vi "N Field Set Act.vi"(0 "command text in":string[](array[string]), 1 "Magnet":T1) -> ()   [LabVIEW 2025]
doc: "Author: Scott Hannahs <sth@magnet.fsu.edu>\n\nThis software is licensed for use under the “MIT License\"\nCopyright (c) 2025 Scott Hannahs, sth@sth@magnet.sthnet.net\n\nPermission is hereby granted, free of charge, to any person obtaining a copy of this software and associated documentation files (the \"Software\"), to deal in the Software without restriction, including without limitation the rights to use, copy, modify, merge, publish, distribute, sublicense, and/or sell copies of the Software, and to permit persons to whom the Software is furnished to do so, subject to the following conditions: The above copyright notice and this permission notice shall be included in all copies or substantial portions of the Software.\n\nTHE SOFTWARE IS PROVIDED \"AS IS\", WITHOUT WARRANTY OF ANY KIND, EXPRESS OR IMPLIED, INCLUDING BUT NOT LIMITED TO THE WARRANTIES OF MERCHANTABILITY, FITNESS FOR A PARTICULAR PURPOSE AND NONINFRINGEMENT. IN NO EVENT SHALL THE AUTHORS OR COPYRIGHT HOLDERS BE LIABLE FOR ANY CLAIM, DAMAGES OR OTHER LIABILITY, WHETHER IN AN ACTION OF CONTRACT, TORT OR OTHERWISE, ARISING FROM, OUT OF OR IN CONNECTION WITH THE SOFTWARE OR THE USE OR OTHER DEALINGS IN THE SOFTWARE."
uses:
  Ctl/magnet.ctl
  Which Power Supply.ctl
panel:
  out "error out 2":errorcluster
  out "error out":errorcluster
  in  "extra wait (sec)":i32
  in  "Rate":dbl
  in  "Field Set":dbl
  # "No wait"
  # "wait"
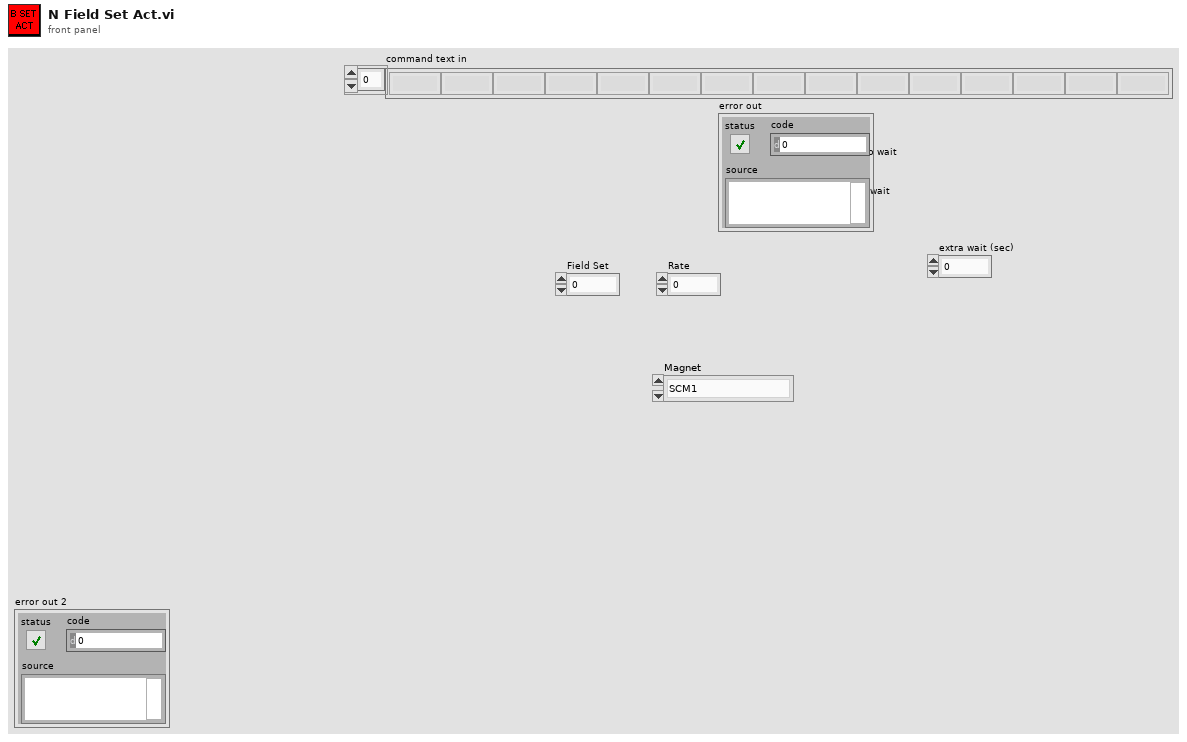
[diagram p1: front panel]
types:
  T1 = typedef "magnet.ctl" = enum16{"SCM1", "SCM2", "SCM3", "SCMX", "Cell8", "Cell9", "Cell12", "Hybrid", "Great Magnet"}
  T2 = typedef "Which Power Supply.ctl" = enum16{"Superconducting Magnet", "Resistive Magnet", "Hybrid Magnet"}
  T3 = typedef "Field Set.ctl" = cluster{"rate":dbl, "set point":dbl, "extra wait":i32, "wait option":u16}
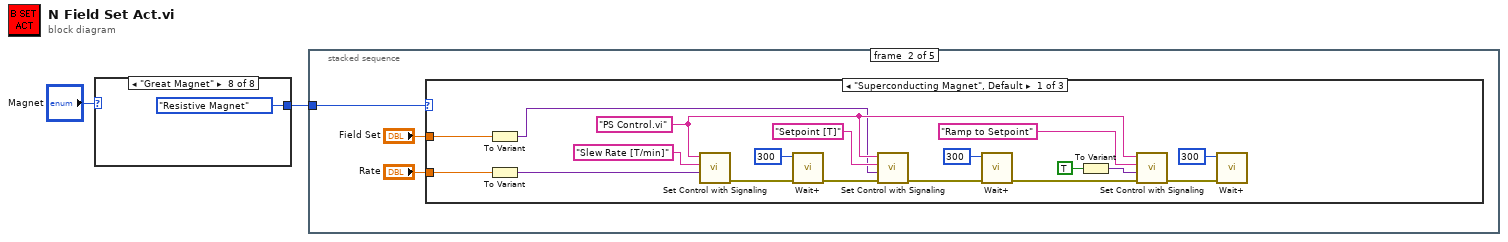
[diagram p0: block diagram]
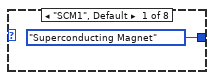
[diagram p2: hidden frame]
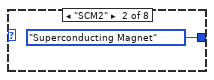
[diagram p3: hidden frame]
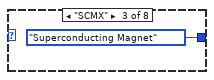
[diagram p4: hidden frame]
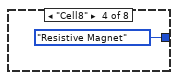
[diagram p5: hidden frame]
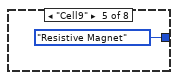
[diagram p6: hidden frame]
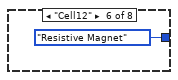
[diagram p7: hidden frame]
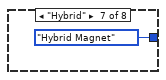
[diagram p8: hidden frame]
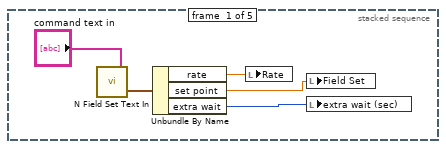
[diagram p9: hidden frame]
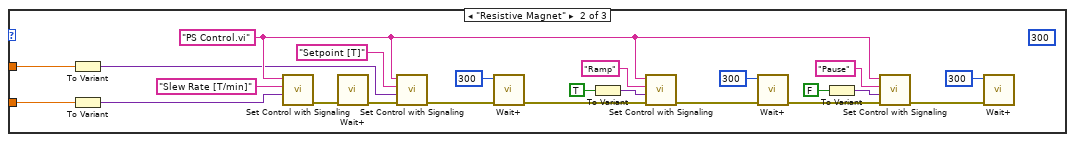
[diagram p10: hidden frame]
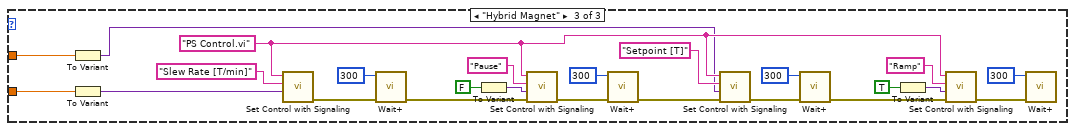
[diagram p11: hidden frame]
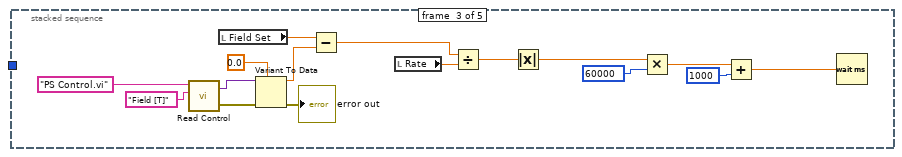
[diagram p12: hidden frame]
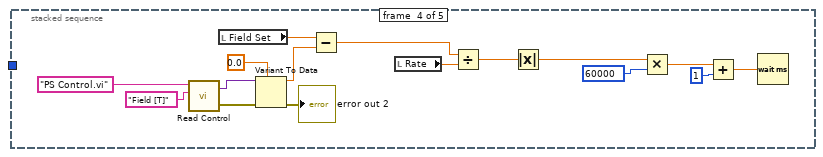
[diagram p13: hidden frame]
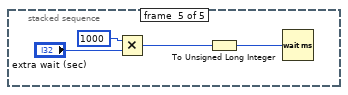
[diagram p14: hidden frame]
diagram:
  n1 = case shown="\"Great Magnet\"" "Magnet" {
    tunnel: [Which_Power_Supply."Superconducting Magnet" ("which power supply") Which_Power_Supply."Superconducting Magnet" ("which power supply") Which_Power_Supply."Superconducting Magnet" ("which power supply") Which_Power_Supply."Resistive Magnet" ("which power supply") Which_Power_Supply."Resistive Magnet" ("which power supply") Which_Power_Supply."Resistive Magnet" ("which power supply") Which_Power_Supply."Hybrid Magnet" ("which power supply") Which_Power_Supply."Resistive Magnet" ("which power supply")] -> w1
    frame "SCM1", Default {
    }
    frame "SCM2" {
    }
    frame "SCMX" {
    }
    frame "Cell8" {
    }
    frame "Cell9" {
    }
    frame "Cell12" {
    }
    frame "Hybrid" {
    }
    frame "Great Magnet" {
    }
  }
  n2 = stacked-sequence {
    tunnel: w1 -> [_ w16 _ _ _]
    frame #0 {
      n3 = call "N Field Set Text In.vi"("command text in"="command text in") -> ("SetFieldCluster"=w15:T3)  [unwired: 4 in]
      n4 = Unbundle By Name(w15) -> ("rate"=w11:dbl, "set point"=w12:dbl, "extra wait"=w13:i32)
      n5 = local write "Rate"(w11) -> ()
      n6 = local write "Field Set"(w12) -> ()
      n7 = local write "extra wait (sec)"(w13) -> ()
    }
    frame #1 {
      n8 = case shown="\"Superconducting Magnet\", Default" w16 {
        tunnel: "Rate" -> [w36 w59 w83]
        tunnel: "Field Set" -> [w35 w58 w82]
        frame "Superconducting Magnet", Default {
          w34 = "PS Control.vi" ("VI name")
          n9 = To Variant(anything=w35) -> (Variant=w24:variant)
          n10 = To Variant(anything=w36) -> (Variant=w27:variant)
          n11 = call "Set Control with Signaling.vi"("Value"=w27, "Control Name"="Slew Rate [T/min]", "VI Name"=w34) -> ("error out"=w33:errorcluster)  [unwired: 8 in]
          n12 = call "Wait+.vi"("Error In"=w33, "milliseconds to wait"=u32 300) -> ("Error Out"=w32:errorcluster)  [unwired: 4 in, 1 out]
          n13 = call "Set Control with Signaling.vi"("error in (no error)"=w32, "Value"=w24, "Control Name"="Setpoint [T]", "VI Name"=w34) -> ("error out"=w31:errorcluster)  [unwired: 7 in]
          n14 = call "Wait+.vi"("Error In"=w31, "milliseconds to wait"=u32 300) -> ("Error Out"=w30:errorcluster)  [unwired: 4 in, 1 out]
          n15 = To Variant(anything=TRUE) -> (Variant=w22:variant)
          n16 = call "Set Control with Signaling.vi"("error in (no error)"=w30, "Value"=w22, "Control Name"="Ramp to Setpoint", "VI Name"=w34) -> ("error out"=w29:errorcluster)  [unwired: 7 in]
          n17 = call "Wait+.vi"("Error In"=w29, "milliseconds to wait"=u32 300) -> ()  [unwired: 4 in, 2 out]
        }
        frame "Resistive Magnet" {
          (unwired) u32 300 ("milliseconds to wait")
          w57 = "PS Control.vi" ("VI name")
          n18 = To Variant(anything=w58) -> (Variant=w46:variant)
          n19 = To Variant(anything=w59) -> (Variant=w48:variant)
          n20 = call "Set Control with Signaling.vi"("Value"=w48, "Control Name"="Slew Rate [T/min]", "VI Name"=w57) -> ("error out"=w56:errorcluster)  [unwired: 8 in]
          n21 = call "Wait+.vi"("Error In"=w56) -> ("Error Out"=w50:errorcluster)  [unwired: 5 in, 1 out]
          n22 = call "Set Control with Signaling.vi"("error in (no error)"=w50, "Value"=w46, "Control Name"="Setpoint [T]", "VI Name"=w57) -> ("error out"=w51:errorcluster)  [unwired: 7 in]
          n23 = call "Wait+.vi"("Error In"=w51, "milliseconds to wait"=u32 300) -> ("Error Out"=w52:errorcluster)  [unwired: 4 in, 1 out]
          n24 = To Variant(anything=TRUE) -> (Variant=w44:variant)
          n25 = call "Set Control with Signaling.vi"("error in (no error)"=w52, "Value"=w44, "Control Name"="Ramp", "VI Name"=w57) -> ("error out"=w53:errorcluster)  [unwired: 7 in]
          n26 = call "Wait+.vi"("Error In"=w53, "milliseconds to wait"=u32 300) -> ("Error Out"=w54:errorcluster)  [unwired: 4 in, 1 out]
          n27 = To Variant(anything=FALSE) -> (Variant=w40:variant)
          n28 = call "Set Control with Signaling.vi"("error in (no error)"=w54, "Value"=w40, "Control Name"="Pause", "VI Name"=w57) -> ("error out"=w55:errorcluster)  [unwired: 7 in]
          n29 = call "Wait+.vi"("Error In"=w55, "milliseconds to wait"=u32 300) -> ()  [unwired: 4 in, 2 out]
        }
        frame "Hybrid Magnet" {
          w81 = "PS Control.vi" ("VI name")
          n30 = To Variant(anything=w82) -> (Variant=w65:variant)
          n31 = To Variant(anything=w83) -> (Variant=w72:variant)
          n32 = call "Set Control with Signaling.vi"("Value"=w72, "Control Name"="Slew Rate [T/min]", "VI Name"=w81) -> ("error out"=w80:errorcluster)  [unwired: 8 in]
          n33 = call "Wait+.vi"("Error In"=w80, "milliseconds to wait"=u32 300) -> ("Error Out"=w79:errorcluster)  [unwired: 4 in, 1 out]
          n34 = To Variant(anything=FALSE) -> (Variant=w70:variant)
          n35 = call "Set Control with Signaling.vi"("error in (no error)"=w79, "Value"=w70, "Control Name"="Pause", "VI Name"=w81) -> ("error out"=w78:errorcluster)  [unwired: 7 in]
          n36 = call "Wait+.vi"("Error In"=w78, "milliseconds to wait"=u32 300) -> ("Error Out"=w77:errorcluster)  [unwired: 4 in, 1 out]
          n37 = call "Set Control with Signaling.vi"("error in (no error)"=w77, "Value"=w65, "Control Name"="Setpoint [T]", "VI Name"=w81) -> ("error out"=w76:errorcluster)  [unwired: 7 in]
          n38 = call "Wait+.vi"("Error In"=w76, "milliseconds to wait"=u32 300) -> ("Error Out"=w75:errorcluster)  [unwired: 4 in, 1 out]
          n39 = To Variant(anything=TRUE) -> (Variant=w63:variant)
          n40 = call "Set Control with Signaling.vi"("error in (no error)"=w75, "Value"=w63, "Control Name"="Ramp", "VI Name"=w81) -> ("error out"=w74:errorcluster)  [unwired: 7 in]
          n41 = call "Wait+.vi"("Error In"=w74, "milliseconds to wait"=u32 300) -> ()  [unwired: 4 in, 2 out]
        }
      }
    }
    frame #2 {
      n42 = call "Read Control.vi"("VI Name"="PS Control.vi", "Control Name"="Field [T]") -> ("Value"=w97:variant, "error out"=w96:errorcluster)  [unwired: 3 in]
      n43 = local read "Field Set"() -> (w86:dbl)
      n44 = Variant To Data(error in=w96, type=0.0 ("Numeric"), Variant=w97) -> (data=w85:dbl, error out=→"error out":errorcluster)
      n45 = Subtract(x=w86, y=w85) -> (x-y=w87:dbl)
      n46 = local read "Rate"() -> (w84:dbl)
      n47 = Divide(x=w87, y=w84) -> (x/y=w88:dbl)
      n48 = Absolute Value(x=w88) -> (abs(x)=w89:dbl)
      n49 = Multiply(x=w89, y=60000) -> (x*y=w92:dbl)
      n50 = Add(x=w92, y=1000) -> (x+y=w93:dbl)
      n51 = Wait (ms)(milliseconds to wait=w93) -> ()  [unwired: 1 out]
    }
    frame #3 {
      n52 = call "Read Control.vi"("VI Name"="PS Control.vi", "Control Name"="Field [T]") -> ("Value"=w102:variant, "error out"=w103:errorcluster)  [unwired: 3 in]
      n53 = local read "Field Set"() -> (w115:dbl)
      n54 = Variant To Data(error in=w103, type=0.0 ("Numeric"), Variant=w102) -> (data=w113:dbl, error out=→"error out 2":errorcluster)
      n55 = Subtract(x=w115, y=w113) -> (x-y=w112:dbl)
      n56 = local read "Rate"() -> (w114:dbl)
      n57 = Divide(x=w112, y=w114) -> (x/y=w111:dbl)
      n58 = Absolute Value(x=w111) -> (abs(x)=w110:dbl)
      n59 = Multiply(x=w110, y=60000) -> (x*y=w107:dbl)
      n60 = Add(x=w107, y=1) -> (x+y=w106:dbl)
      n61 = Wait (ms)(milliseconds to wait=w106) -> ()  [unwired: 1 out]
    }
    frame #4 {
      n62 = Multiply(x=1000 ("y"), y="extra wait (sec)") -> (x*y=w117:i32)
      n63 = To Unsigned Long Integer(number=w117) -> (unsigned 32bit integer=w116:u32)
      n64 = Wait (ms)(milliseconds to wait=w116) -> ()  [unwired: 1 out]
    }
  }
